vi "Find Control Set from Control Reference.vi"(2 "error in (no error)":errorcluster, 3 "Control Set Array":refnum<vi>[][](array[refnum]), 4 "Control to Search For":refnum<vi>) -> (0 "error out":errorcluster, 1 "Index":i32)   [LabVIEW 2020]
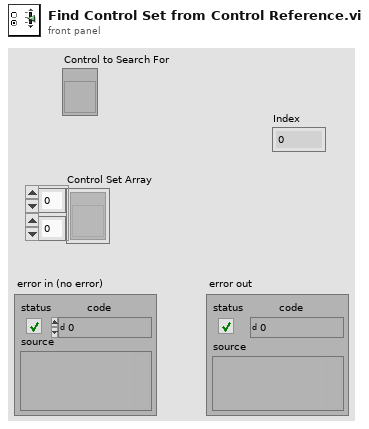
[diagram p1: front panel]
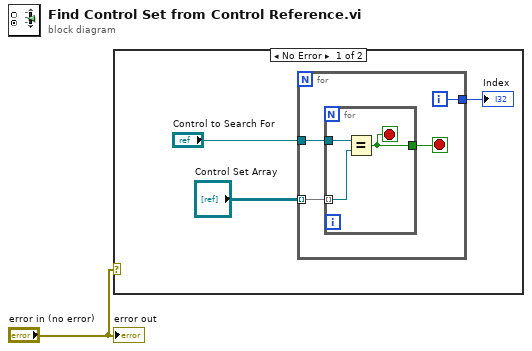
[diagram p0: block diagram]
diagram:
  n1 = case shown="No Error" "error in (no error)" {
    frame No Error {
      n2 = for {
        tunnel: "Control to Search For" -> [w7]
        tunnel: [w8] -> w3
        tunnel: "Control Set Array" -> [w6] mode=indexing
        i -> [w8]
        stop <- w5 stop-if-true
        n3 = for {
          tunnel: w7 -> [w11]
          tunnel: w6 -> [w10] mode=indexing
          tunnel: [w9] -> w5
          stop <- w9 stop-if-true
          n4 = Equal?(x=w11, y=w10) -> (x = y?=w9:bool)
        }
      }
      "Index" <- w3
    }
    frame Error {
    }
  }
  "error out" <- "error in (no error)"
